vi "testEscapeChars.vi"(8 "error in (no error)":errorcluster, 11 "reference in":refnum<class "EasyXMLTest.lvclass">) -> (0 "error out":errorcluster, 3 "reference in":refnum<class "EasyXMLTest.lvclass">)   [LabVIEW 2011, in "EasyXMLTest.lvclass"]
uses:
  EasyXMLTest.lvclass
panel:
  in  "XML String":string="<Escape_Chars>\r\n  <Char>&amp;</Char>\r\n  <Char>&gt;</Char>\r\n  <Char>&lt;</Char>\r\n</Escape_Chars>"
  in  "Escape Chars":cluster{"Char":string[]}={"Char"=["&", ">", "<"]}
  out "Generated XML String":string
  out "Produced Data":cluster{"Char":string[]}
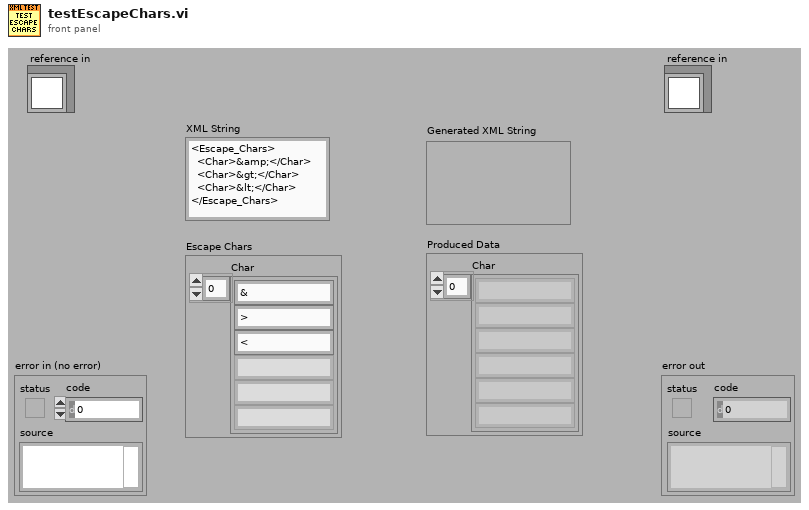
[diagram p1: front panel]
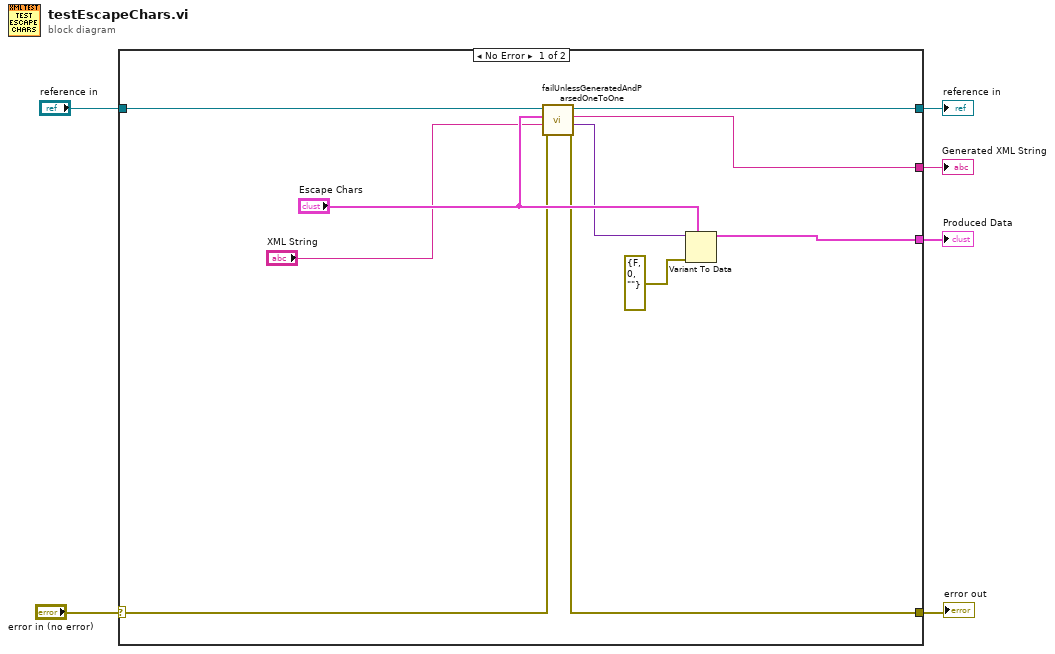
[diagram p0: block diagram]
diagram:
  n1 = case shown="No Error" "error in (no error)" {
    selector: "error in (no error)" -> [w10 w18]
    tunnel: [w9 w18] -> w5
    tunnel: [w13 w17] -> w3
    tunnel: "reference in" -> [w14 w17]
    tunnel: [w8 _] -> w2
    tunnel: [w16 _] -> w1
    frame No Error {
      n2 = call "failUnlessGeneratedAndParsedOneToOne.vi"("error in"=w10, "XML String"="XML String", "Data"="Escape Chars", "EasyXMLTest in"=w14) -> ("error out"=w9:errorcluster, "Produced Data"=w7:variant, "Generated XML String"=w8:string, "EasyXMLTest out"=w13:refnum<class "EasyXMLTest.lvclass">)  [unwired: 4 in]
      n3 = Variant To Data(error in=errorcluster {"status"=FALSE, "code"=0, "source"=""}, type="Escape Chars", Variant=w7) -> (data=w16:cluster{"Char":string[]})  [unwired: 1 out]
    }
    frame Error {
    }
  }
  "error out" <- w5
  "reference in" <- w3
  "Generated XML String" <- w2
  "Produced Data" <- w1
